vi "GSP_Manager_Mode.vi"() -> ()   [LabVIEW 2015]
uses:
  SystemUtil/Command.ctl
  Wavelength/movetypes.ctl
  Wavelength/wavelength_parameters.ctl
  GSCS Scripting/Utils/GSP_Wavelength_Global.vi
  Grating_Translation/GSP_GT_Global.vi
  SystemUtil/ThreadStates.ctl
panel:
  in  "Grating Angle Target":dbl
  in  "Previous Grating Angle":dbl
  in  "Previous Camera Angle":dbl
  in  "Camera Target":dbl
  in  "Grating Target":i32
  in  "Previous Grating":i32
  out "Imaging":bool
  in  "Image Slit":bool
  out "Last Error":errorcluster
  in  "CommandQ":string
  # "Mask Imaging"
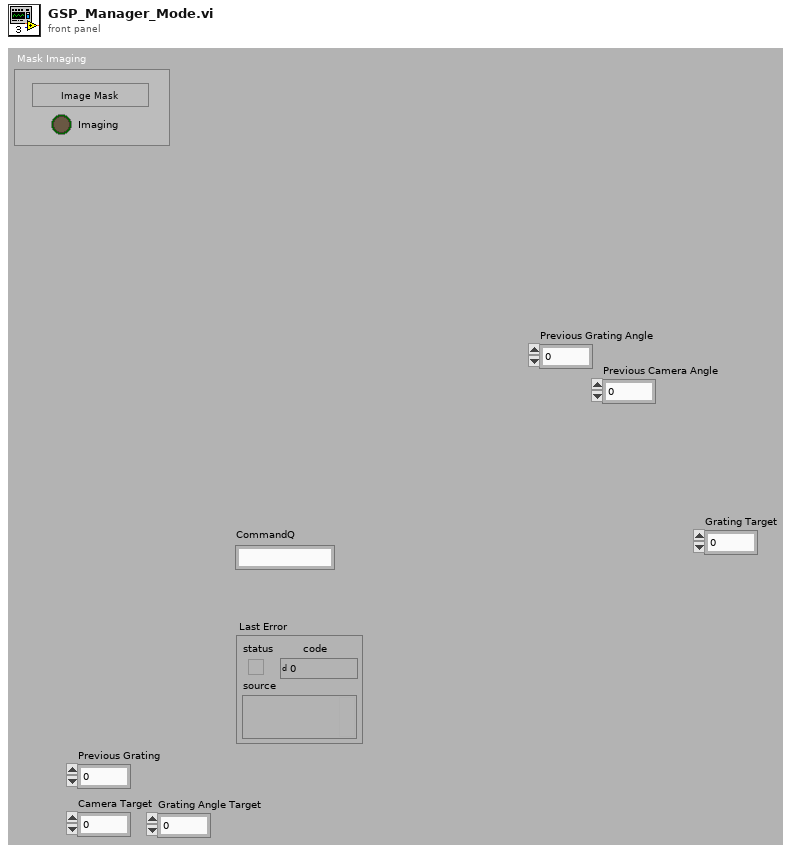
[diagram p1: front panel]
types:
  T1 = typedef "Command.ctl" = cluster{"Command":string, "Parameter":string}
  T2 = typedef "ThreadStates.ctl" = enum16{"Waiting", "Scripting", "Uninitialized", "Error"}
  T3 = typedef "wavelength_parameters.ctl" = cluster{"Camera Angle":dbl, "Grating  Angle":dbl, "Move type":T4}
  T4 = typedef "movetypes.ctl" = u16
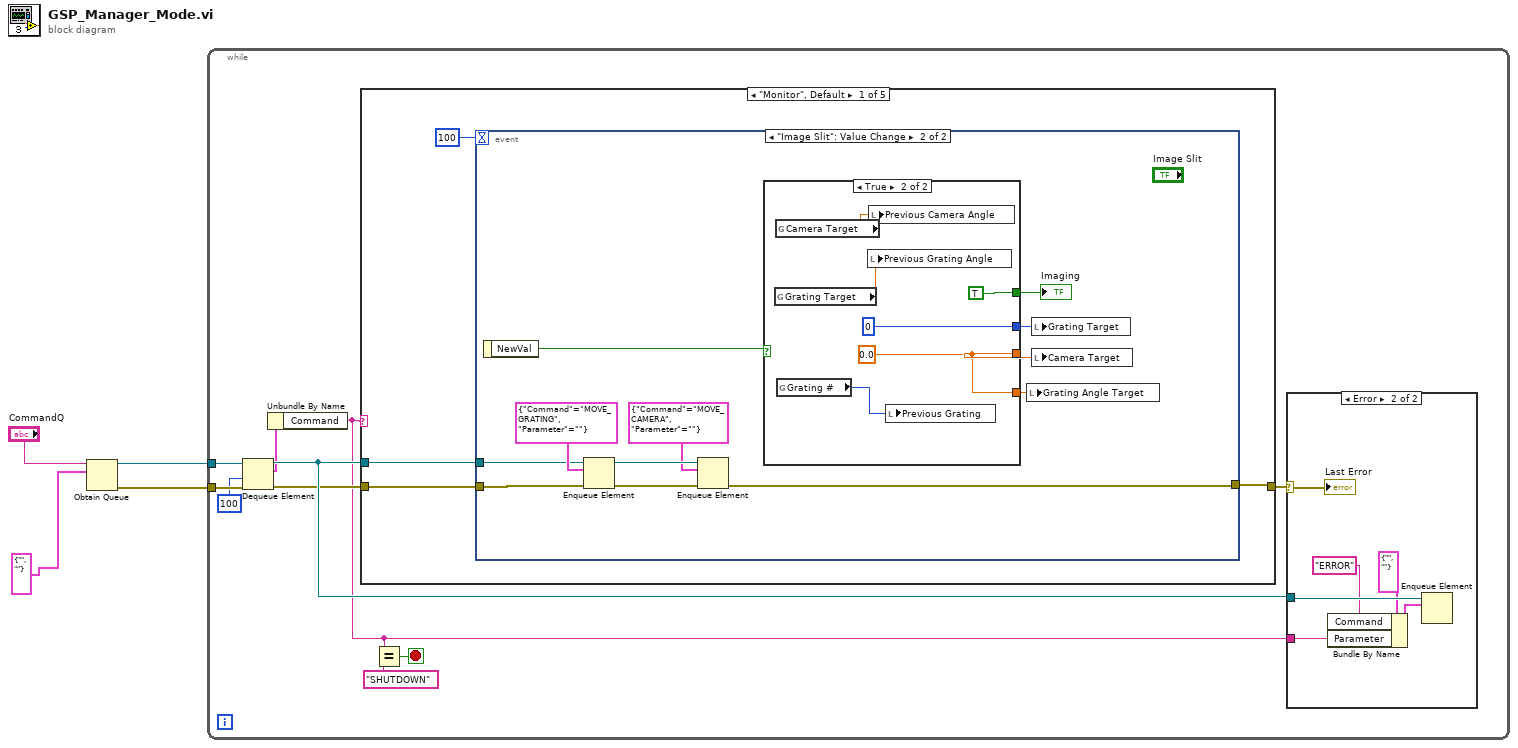
[diagram p0: block diagram]
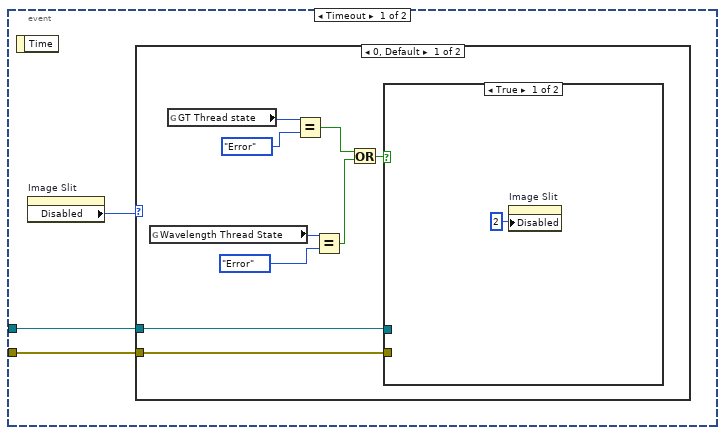
[diagram p3: hidden frame]
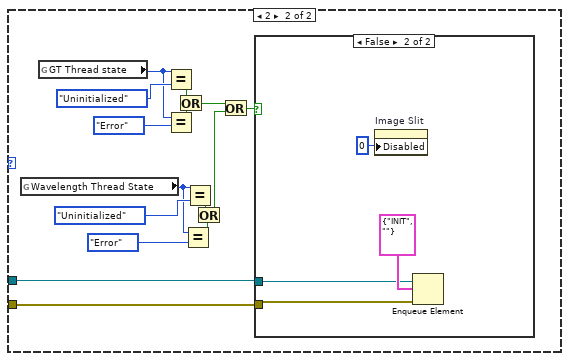
[diagram p5: hidden frame]
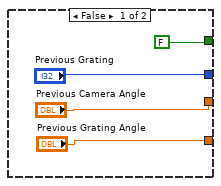
[diagram p7: hidden frame]
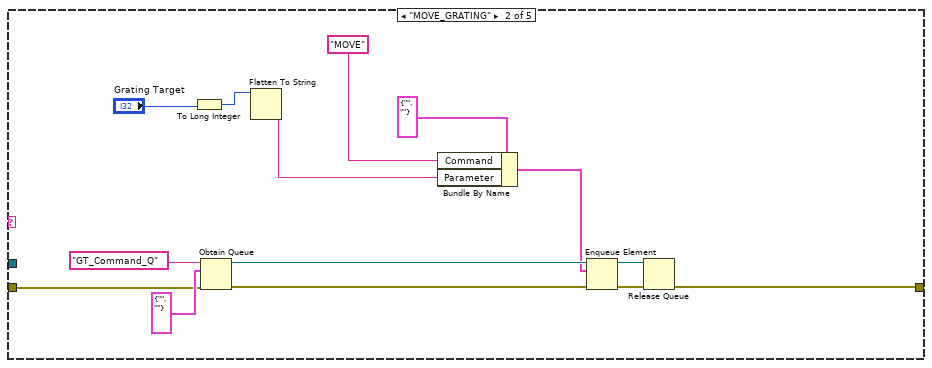
[diagram p8: hidden frame]
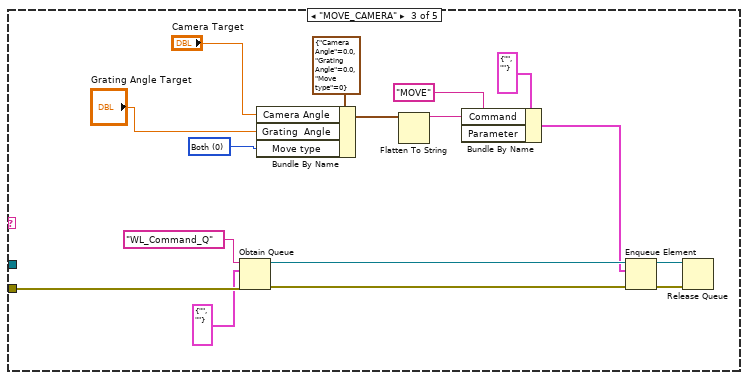
[diagram p9: hidden frame]
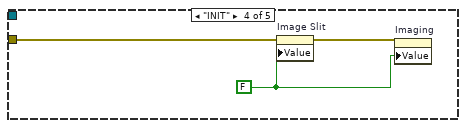
[diagram p10: hidden frame]
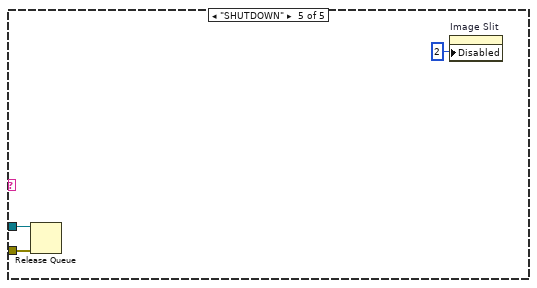
[diagram p11: hidden frame]
diagram:
  n1 = Obtain Queue(name (unnamed)="CommandQ", element data type=T1 {"Command"="", "Parameter"=""} ("Command")) -> (queue out=w2:refnum<queue>, error out=w1:errorcluster)  [unwired: 3 in, 1 out]
  n2 = while {
    tunnel: w2 -> [w14]
    tunnel: w1 -> [w13]
    stop <- w6 stop-if-true
    n3 = Dequeue Element(queue=w14, timeout in ms (-1)=100, error in (no error)=w13) -> (queue out=w11:refnum<queue>, element=w7:T1, error out=w9:errorcluster)  [unwired: 1 out]
    n4 = Unbundle By Name(w7) -> ("Command"=w5:string)
    n5 = case shown="\"Monitor\", Default" w5 {
      tunnel: w9 -> [w23 w84 w104 w111 w114]
      tunnel: w11 -> [w24 _ _ _ w113]
      tunnel: [w22 w80 _ _ _] -> w12
      frame "Monitor", Default {
        n6 = event shown="[1] \"Image Slit\": Value Change" {
          selector: _ -> [_ _]
          dyn-events: _ -> [_ _]
          timeout: 100 -> [_ _]
          tunnel: w24 -> [w25 w63]
          tunnel: w23 -> [w27 w62]
          tunnel: [_ w61] -> w22
          event Timeout {
            n7 = event-data() -> ()  [unwired: 1 in, 1 out]
            n8 = property on="Image Slit" class="Bool (strict)"() -> ("Disabled"=w26:u8)  [unwired: 2 in, 2 out]
            n9 = case shown="0, Default" w26 {
              tunnel: w27 -> [w30 w52]
              tunnel: w25 -> [w31 w51]
              frame 0, Default {
                n10 = global read "GSP_Wavelength_Global.vi" "Wavelength Thread State"() -> (w33:T2)
                n11 = global read "GSP_GT_Global.vi" "GT Thread state"() -> (w35:T2)
                n12 = Equal?(x=w35, y=ThreadStates."Error" ("GT Thread state")) -> (x = y?=w29:bool)
                n13 = Equal?(x=w33, y=ThreadStates."Error" ("Wavelength Thread State")) -> (x = y?=w28:bool)
                n14 = Or(x=w29, y=w28) -> (x .or. y?=w32:bool)
                n15 = case shown="True" w32 {
                  tunnel: w30 -> [_ _]
                  tunnel: w31 -> [_ _]
                  frame True {
                    n16 = property on="Image Slit" class="Bool (strict)"("Disabled"=u8 2) -> ()  [unwired: 2 in, 2 out]
                  }
                  frame False {
                  }
                }
              }
              frame 2 {
                n17 = global read "GSP_Wavelength_Global.vi" "Wavelength Thread State"() -> (w43:T2)
                n18 = global read "GSP_GT_Global.vi" "GT Thread state"() -> (w47:T2)
                n19 = Equal?(x=w47, y=ThreadStates."Uninitialized" ("GT Thread state")) -> (x = y?=w50:bool)
                n20 = Equal?(x=w47, y=ThreadStates."Error" ("GT Thread state")) -> (x = y?=w48:bool)
                n21 = Or(x=w50, y=w48) -> (x .or. y?=w39:bool)
                n22 = Equal?(x=w43, y=ThreadStates."Error" ("Wavelength Thread State")) -> (x = y?=w41:bool)
                n23 = Equal?(x=w43, y=ThreadStates."Uninitialized" ("Wavelength Thread State")) -> (x = y?=w44:bool)
                n24 = Or(x=w44, y=w41) -> (x .or. y?=w40:bool)
                n25 = Or(x=w39, y=w40) -> (x .or. y?=w38:bool)
                n26 = case shown="False" w38 {
                  tunnel: w52 -> [_ w55]
                  tunnel: w51 -> [_ w54]
                  frame True {
                  }
                  frame False {
                    n27 = property on="Image Slit" class="Bool (strict)"("Disabled"=u8 0) -> ()  [unwired: 2 in, 2 out]
                    n28 = Enqueue Element(queue=w54, element=T1 {"Command"="INIT", "Parameter"=""} ("Command"), error in (no error)=w55) -> ()  [unwired: 1 in, 3 out]
                  }
                }
              }
            }
          }
          event "Image Slit": Value Change {
            n29 = event-data() -> ("NewVal"=w68:bool)  [unwired: 1 in]
            n30 = Enqueue Element(queue=w63, element=T1 {"Command"="MOVE_GRATING", "Parameter"=""} ("Command"), error in (no error)=w62) -> (queue out=w67:refnum<queue>, error out=w66:errorcluster)  [unwired: 1 in, 1 out]
            n31 = Enqueue Element(queue=w67, element=T1 {"Command"="MOVE_CAMERA", "Parameter"=""} ("Command"), error in (no error)=w66) -> (error out=w61:errorcluster)  [unwired: 1 in, 2 out]
            n32 = case shown="True" w68 {
              tunnel: [FALSE ("Imaging") TRUE ("Imaging")] -> w60
              tunnel: ["Previous Grating" 0 ("Grating Target")] -> w59
              tunnel: ["Previous Camera Angle" w73] -> w58
              tunnel: ["Previous Grating Angle" w73] -> w57
              frame False {
              }
              frame True {
                w73 = 0.0 ("Camera Target")
                n33 = global read "GSP_Wavelength_Global.vi" "Grating Target"() -> (w74:dbl)
                n34 = global read "GSP_Wavelength_Global.vi" "Camera Target"() -> (w76:dbl)
                n35 = global read "GSP_GT_Global.vi" "Grating #"() -> (w75:i32)
                n36 = local write "Previous Grating Angle"(w74) -> ()
                n37 = local write "Previous Camera Angle"(w76) -> ()
                n38 = local write "Previous Grating"(w75) -> ()
              }
            }
            "Imaging" <- w60
            n39 = local write "Grating Angle Target"(w57) -> ()
            n40 = local write "Grating Target"(w59) -> ()
            n41 = local write "Camera Target"(w58) -> ()
          }
        }
      }
      frame "MOVE_GRATING" {
        n42 = To Long Integer(number="Grating Target") -> (32bit integer=w89:i32)
        n43 = Obtain Queue(name (unnamed)="GT_Command_Q", element data type=T1 {"Command"="", "Parameter"=""} ("Command"), error in (no error)=w84) -> (queue out=w85:refnum<queue>, error out=w83:errorcluster)  [unwired: 2 in, 1 out]
        n44 = Flatten To String(anything=w89) -> (data string=w90:string)  [unwired: 3 in, 2 out]
        n45 = Bundle By Name(cluster=T1 {"Command"="", "Parameter"=""} ("Command"), "Command"="MOVE" ("element"), "Parameter"=w90) -> (w79:T1)
        n46 = Enqueue Element(queue=w85, element=w79, error in (no error)=w83) -> (queue out=w82:refnum<queue>, error out=w81:errorcluster)  [unwired: 1 in, 1 out]
        n47 = Release Queue(queue=w82, error in (no error)=w81) -> (error out=w80:errorcluster)  [unwired: 1 in, 2 out]
      }
      frame "MOVE_CAMERA" {
        w95 = T4 0 items=["Both", "Grating Only", "Camera Only"] ("Move type")
        n48 = Obtain Queue(name (unnamed)="WL_Command_Q", element data type=T1 {"Command"="", "Parameter"=""} ("Command"), error in (no error)=w104) -> (queue out=w108:refnum<queue>, error out=w107:errorcluster)  [unwired: 2 in, 1 out]
        n49 = Bundle By Name(cluster=T3 {"Camera Angle"=0.0, "Grating  Angle"=0.0, "Move type"=0} ("Wavelength Parameters"), "Camera Angle"="Camera Target", "Grating  Angle"="Grating Angle Target", "Move type"=w95) -> (w97:T3)
        n50 = Flatten To String(anything=w97) -> (data string=w100:string)  [unwired: 3 in, 2 out]
        n51 = Bundle By Name(cluster=T1 {"Command"="", "Parameter"=""} ("element"), "Command"="MOVE", "Parameter"=w100) -> (w96:T1)
        n52 = Enqueue Element(queue=w108, element=w96, error in (no error)=w107) -> (queue out=w106:refnum<queue>, error out=w105:errorcluster)  [unwired: 1 in, 1 out]
        n53 = Release Queue(queue=w106, error in (no error)=w105) -> ()  [unwired: 1 in, 3 out]
      }
      frame "INIT" {
        w109 = FALSE ("Image Slit")
        n54 = property on="Image Slit" class="Bool (strict)"(error in=w111, "Value"=w109) -> (error out=w110:errorcluster)  [unwired: 1 in, 1 out]
        n55 = property on="Imaging" class="Bool (strict)"(error in=w110, "Value"=w109) -> ()  [unwired: 1 in, 2 out]
      }
      frame "SHUTDOWN" {
        n56 = Release Queue(queue=w113, error in (no error)=w114) -> ()  [unwired: 1 in, 3 out]
        n57 = property on="Image Slit" class="Bool (strict)"("Disabled"=u8 2) -> ()  [unwired: 2 in, 2 out]
      }
    }
    n58 = Equal?(x=w5, y="SHUTDOWN") -> (x = y?=w6:bool)
    n59 = case shown="Error" w12 {
      selector: w12 -> [_ w19]
      tunnel: w11 -> [_ w20]
      tunnel: w5 -> [_ w16]
      frame No Error {
      }
      frame Error {
        n60 = Bundle By Name(cluster=T1 {"Command"="", "Parameter"=""} ("element"), "Command"="ERROR" ("element"), "Parameter"=w16) -> (w18:T1)
        n61 = Enqueue Element(queue=w20, element=w18) -> ()  [unwired: 2 in, 3 out]
        "Last Error" <- w19
      }
    }
  }
